vi "Get 2D Array Double.vi"(5 "use temporary file? (F)":bool, 7 "data type of variable":dbl[][](array[numeric]), 8 "error in":errorcluster, 10 "variable name":string, 11 "GOLPI ref. in":T1={"pipe handle"={"lv_proc.dll file path"=path "", "process instance handle"=[], "debug mode"=FALSE, "debug data"=[]}, "fast read timeout [ms]"=500, "fast read settle time [ms]"=10, "fast read to multiple [ms]"=1, "max elements per input line"=100, "slow read timeout [ms]"=5000, "stdin double format specifier"="%_16e", "max elements per stdout output column"=100, "console mode bitstream"=FALSE, "bitstream first read timeout [ms]"=1000, "bitstream read timeout [ms]"=50, "struct transfer possible"=FALSE, "matlab mode"=FALSE, "var pipe write timeout [ms]"=5000, "variable pipe mode"=FALSE, "variable pipe buffer size [Bytes]"=10000000, "variable pipe block size [Bytes]"=1000000} {"variable pipe block size [Bytes]" format="%.0p"; "variable pipe buffer size [Bytes]" format="%.0p"}) -> (0 "error out":errorcluster, 2 "value":dbl[][](array[numeric]) format="%.2f", 3 "GOLPI ref. out":T1={"pipe handle"={"lv_proc.dll file path"=path "", "process instance handle"=[], "debug mode"=FALSE, "debug data"=[]}, "fast read timeout [ms]"=500, "fast read settle time [ms]"=10, "fast read to multiple [ms]"=1, "max elements per input line"=100, "slow read timeout [ms]"=5000, "stdin double format specifier"="%_16e", "max elements per stdout output column"=100, "console mode bitstream"=FALSE, "bitstream first read timeout [ms]"=1000, "bitstream read timeout [ms]"=50, "struct transfer possible"=FALSE, "matlab mode"=FALSE, "var pipe write timeout [ms]"=5000, "variable pipe mode"=FALSE, "variable pipe buffer size [Bytes]"=10000000, "variable pipe block size [Bytes]"=1000000} {"variable pipe block size [Bytes]" format="%.0p"; "variable pipe buffer size [Bytes]" format="%.0p"})   [LabVIEW 2020, in "GOLPI library.lvlib"]
doc: "Part of polymorph Get Variable.vi"
uses:
  GOLPI library.lvlib
  Public/GOLPI reference Type Def.ctl
  LV Process source distribution/Pipe Handle.ctl
  Type Definitions/Bitstream Data Type.ctl
  Type Definitions/Custom Error Codes Enum Type Def.vi
  LV Process source distribution/LV Process library.lvlib
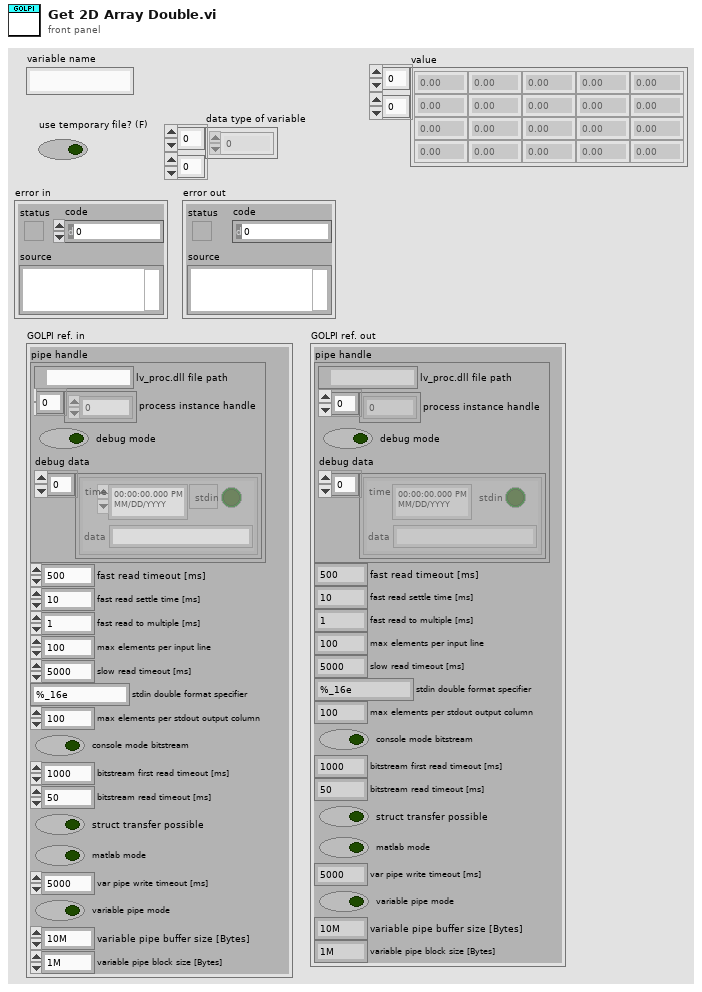
[diagram p1: front panel]
types:
  T1 = typedef "GOLPI library.lvlib/GOLPI reference Type Def.ctl" = cluster{"pipe handle":T2, "fast read timeout [ms]":u32, "fast read settle time [ms]":u32, "fast read to multiple [ms]":u32, "max elements per input line":u32, "slow read timeout [ms]":u32, "stdin double format specifier":string, "max elements per stdout output column":u32, "console mode bitstream":bool, "bitstream first read timeout [ms]":u32, "bitstream read timeout [ms]":u32, "struct transfer possible":bool, "matlab mode":bool, "var pipe write timeout [ms]":u32, "variable pipe mode":bool, "variable pipe buffer size [Bytes]":u32, "variable pipe block size [Bytes]":u32}
  T2 = typedef "LV Process library.lvlib/Pipe Handle.ctl" = cluster{"lv_proc.dll file path":path, "process instance handle":u32[], "debug mode":bool, "debug data":cluster{"time":timestamp, "stdin":bool, "data":string}[]}
  T3 = typedef "GOLPI library.lvlib/Custom Error Codes Enum Type Def.vi" = enum16{"no error", "00 working directory PAR1 missing", "01 octave binary PAR1 missing", "02 octave report error PAR1", "03 empty output last cmd PAR1", "04 missing temporary file PAR1", "05 pwd PAR 1 not exist", "06 oct package not installed", "07 octave default binary missing", "10 var PAR1 not string, vect", "11 var PAR1 not num, scal, ~compl", "12 var PAR1 not num, scal, compl", "13 var PAR1 not num, vect, ~compl", "14 var PAR1 not num, vect, compl", "15 var PAR1 not num, mat, ~compl", "16 var PAR1 not num, mat, ~compl", "30 read timeout", "60 bitstream transport failed", "61 bitstream decode error PAR1", "62 bitstream cannot be set", "70 struct transfer not possible", "80 struct: cluster elem. PAR1 not implem.", "81 struct: structure field PAR1 not implem.", "82 struct: size mismatch of PAR1", "83 struct: type mismatch of PAR1", "98 internal error", "99 not finished", "90 Not supported in Matlab mode", "91 Matlab variable transfer error", "92 Matlab Script Error"}
  T4 = typedef "GOLPI library.lvlib/Bitstream Data Type.ctl" = enum16{"dummy", "int", "uint", "float", "complex", "str", "real numeric"}
  T5 = typedef "GOLPI library.lvlib/Transfer Mode.ctl" = enum16{"Matlab", "stdio", "temp file", "bitstream", "pipe"}
  T6 = typedef "GOLPI library.lvlib/Bitstream Data.ctl" = cluster{"double":dbl[][], "cplx double":cdb[][], "int64":i64[][], "uint64":u64[][], "str":string[], "data type":T4}
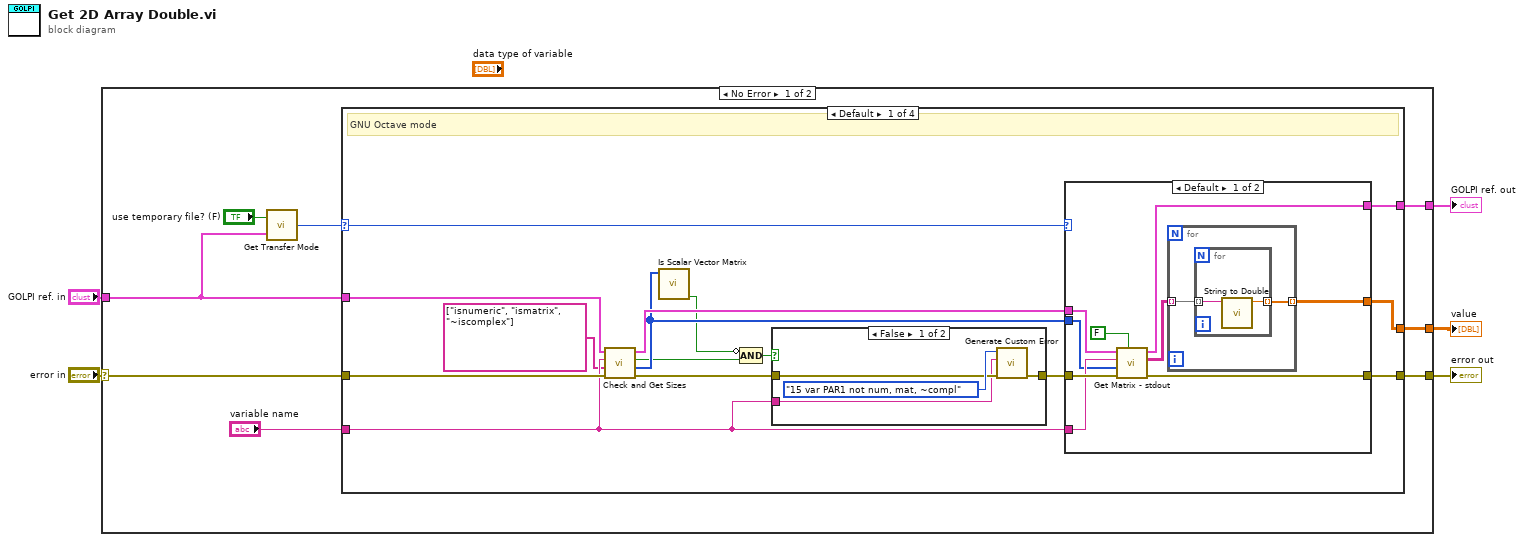
[diagram p0: block diagram]
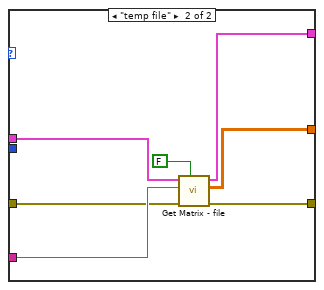
[diagram p2: hidden frame]
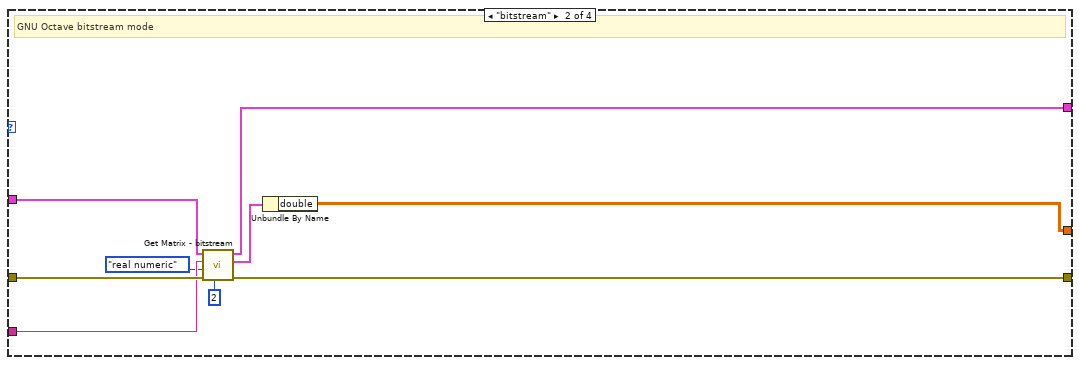
[diagram p4: hidden frame]
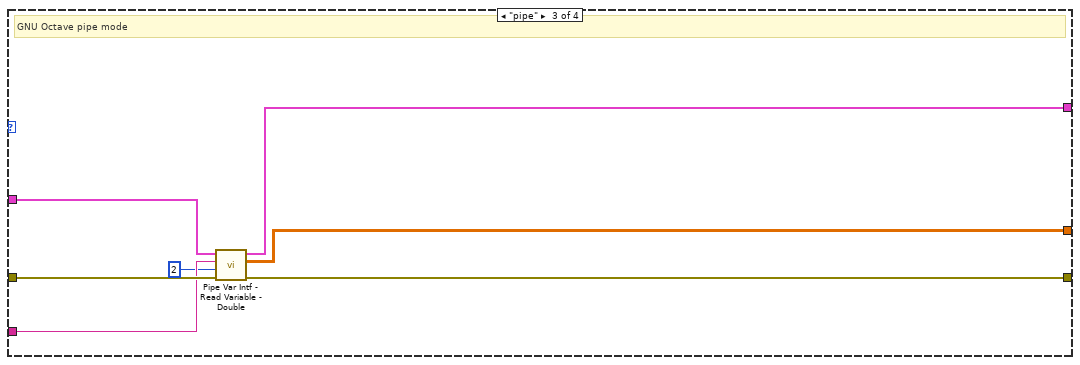
[diagram p5: hidden frame]
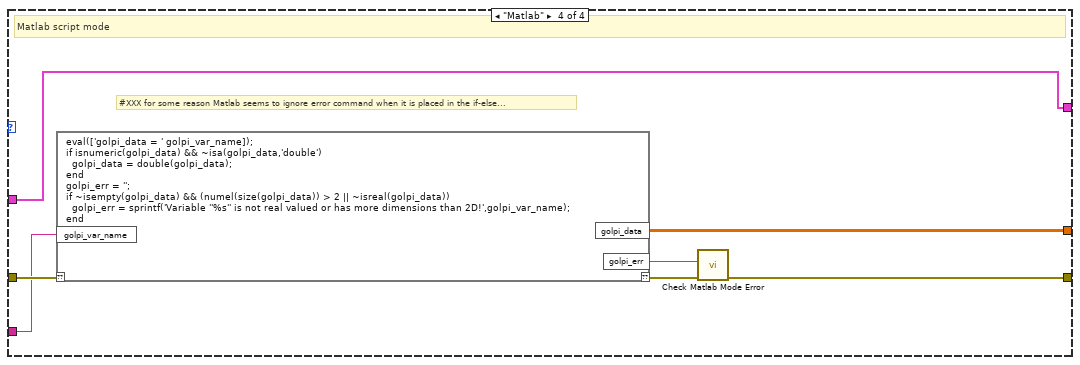
[diagram p6: hidden frame]
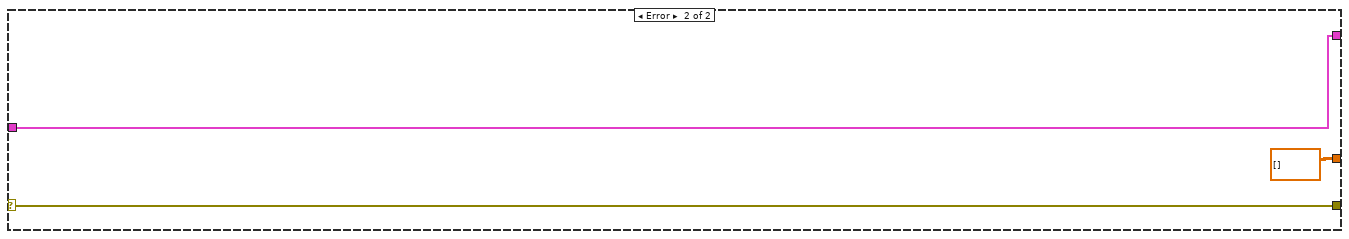
[diagram p7: hidden frame]
diagram:
  n1 = case shown="No Error" "error in" {
    selector: "error in" -> [w12 w79]
    tunnel: [w11 w79] -> w5
    tunnel: [w13 dbl[][] [] ("double array")] -> w3
    tunnel: "GOLPI ref. in" -> [w8 w77]
    tunnel: [w9 w77] -> w1
    frame No Error {
      n2 = call "Get Transfer Mode.vi"("GOLPI ref."=w8, "use temporary file? (F)"="use temporary file? (F)") -> ("mode"=w6:T5)
      n3 = case shown="Default" w6 {
        selector: w6 -> [w14 _ _ _]
        tunnel: [w28 w62 w63 w73] -> w13
        tunnel: w12 -> [w27 w61 w69 w76]
        tunnel: [w26 w60 w68 w70] -> w11
        tunnel: "variable name" -> [w25 w59 w65 w75]
        tunnel: [w24 w58 w66 w74] -> w9
        tunnel: w8 -> [w23 w57 w67 w74]
        frame Default {
          # "GNU Octave mode"
          n4 = call "Check and Get Sizes.vi"("error in (no error)"=w27, "test commands"=string[] ["isnumeric", "ismatrix", "~iscomplex"], "variable name"=w25, "GOLPI ref. in"=w23) -> ("error out"=w22:errorcluster, "octave sizes"=w18:i32[], "all tests OK?"=w16:bool, "GOLPI ref. out"=w20:T1)  [unwired: 4 in]
          n5 = call "Is Scalar Vector Matrix.vi"("octave sizes"=w18) -> ("is >2d matrix?"=w15:bool)  [unwired: 5 in, 5 out]
          n6 = Compound Arithmetic op=AND(invert w15, w16) -> (w17:bool)
          n7 = case shown="False" w17 {
            tunnel: w22 -> [w51 w53]
            tunnel: [w50 w53] -> w19
            tunnel: w25 -> [w49 _]
            frame False {
              n8 = call "Generate Custom Error.vi"("error in"=w51, "PAR1"=w49, "GOLPI error"=Custom_Error_Codes_Enum_Type_Def.vi."15 var PAR1 not num, mat, ~compl" ("Enum")) -> ("error out"=w50:errorcluster)  [unwired: 8 in]
            }
            frame True {
            }
          }
          n9 = case shown="Default" w14 {
            tunnel: [w29 w42] -> w28
            tunnel: w20 -> [w34 w47]
            tunnel: [w31 w46] -> w24
            tunnel: w19 -> [w37 w44]
            tunnel: [w36 w43] -> w26
            tunnel: w25 -> [w35 w45]
            tunnel: w18 -> [w32 _]
            frame Default {
              n10 = call "Get Matrix - stdout.vi"("is string?"=FALSE ("is string"), "error in (no error)"=w37, "octave sizes"=w32, "variable name"=w35, "GOLPI ref. in"=w34) -> ("error out"=w36:errorcluster, "array"=w30:string[][], "GOLPI ref. out"=w31:T1)  [unwired: 4 in]
              n11 = for {
                tunnel: w30 -> [w39] mode=indexing
                tunnel: [w38] -> w29 mode=indexing
                n12 = for {
                  tunnel: w39 -> [w41] mode=indexing
                  tunnel: [w40] -> w38 mode=indexing
                  n13 = call "String to Double.vi"("string"=w41) -> ("number"=w40:dbl)  [unwired: 10 in]
                }
              }
            }
            frame "temp file" {
              n14 = call "Get Matrix - file.vi"("is string?"=FALSE ("is string"), "error in (no error)"=w44, "variable name"=w45, "GOLPI ref. in"=w47) -> ("error out"=w43:errorcluster, "double array"=w42:dbl[][], "GOLPI ref. out"=w46:T1)  [unwired: 3 in, 2 out]
            }
          }
        }
        frame "bitstream" {
          # "GNU Octave bitstream mode"
          n15 = call "Get Matrix - bitstream.vi"("max dimensions (0: scalar)"=2, "error in (no error)"=w61, "data type"=Bitstream_Data_Type."real numeric", "variable name"=w59, "GOLPI ref. in"=w57) -> ("error out"=w60:errorcluster, "data"=w54:T6, "GOLPI ref. out"=w58:T1)  [unwired: 4 in]
          n16 = Unbundle By Name(w54) -> ("double"=w62:dbl[][])
        }
        frame "pipe" {
          # "GNU Octave pipe mode"
          n17 = call "Pipe Var Intf - Read Variable - Double.vi"("error in (no error)"=w69, "max dims (0: scalar)"=2 ("max dimensions (0: scalar)"), "variable name"=w65, "GOLPI ref. in"=w67) -> ("error out"=w68:errorcluster, "data out"=w63:dbl[][], "GOLPI ref. out"=w66:T1)  [unwired: 5 in]
        }
        frame "Matlab" {
          # "#XXX for some reason Matlab seems to ignore error command when it is placed in the if-else..."
          # "Matlab script mode"
          n18 = script code="eval(['golpi_data = ' golpi_var_name]);\nif isnumeric(golpi_data) && ~isa(golpi_data,'double')\n  golpi_data = double(golpi_data);\nend\ngolpi_err = '';\nif ~isempty(golpi_data) && (numel(size(golpi_data)) > 2 || ~isreal(golpi_data))\n  golpi_err = sprintf('Variable ''%s'' is not real valued or has more dimensions than 2D!',golpi_var_name);\nend"("??"=w76, "golpi_var_name"=w75) -> ("??"=w72:errorcluster, "golpi_data"=w73:dbl[][], "golpi_err"=w71:string)
          n19 = call "Check Matlab Mode Error.vi"("error in"=w72, "custom error string (empty)"=w71) -> ("error out"=w70:errorcluster)  [unwired: 9 in]
        }
      }
    }
    frame Error {
    }
  }
  "value" <- w3
  "error out" <- w5
  "GOLPI ref. out" <- w1
